vi "NewFile.vi"(8 "error in (no error)":errorcluster, 9 "data flow":T13, 10 "data event in":T17, 11 "config":T22) -> (0 "error out":errorcluster, 2 "data event out":T17, 3 "data event":T1, 4 "registry":T9, 5 "save waveforms":bool)   [LabVIEW 2017, in "McsaDataEventCreator.lvlib"]
uses:
  <vilib>/addons/InsightCM/Devices/Shared/Mcsa/McsaDataEventCreator/McsaDataEventCreator.lvlib
  <vilib>/addons/InsightCM/Devices/Shared/Mcsa/McsaDataEventCreator/controls/config.ctl
  <vilib>/addons/InsightCM/Devices/Shared/Mcsa/McsaDataEventCreator/controls/DataEventConfig.ctl
  <vilib>/addons/InsightCM/Devices/Shared/Mcsa/McsaDataEventCreator/controls/AcqParams.ctl
  <vilib>/addons/InsightCM/Devices/Shared/Common/DataAccumulator/controls/AccumulationSettings.ctl
  <vilib>/addons/InsightCM/Devices/Shared/Common/DataAccumulator/controls/accumulationType.ctl
  <vilib>/addons/InsightCM/Devices/Shared/Common/DVRBuffer/controls/BufferLocation.ctl
  <vilib>/addons/PointValueMap/controls/PointMap.ctl
  <vilib>/addons/InsightCM/Devices/Shared/Common/DataFlow/controls/Data.ctl
  <vilib>/addons/InsightCM/Utilities/DataAccessors/controls/wfmSGL_DVR.ctl
  <vilib>/addons/InsightCM/Devices/Shared/Common/DataFlow/controls/Type.ctl
  <vilib>/addons/InsightCM/Devices/Shared/Mcsa/McsaDataEventCreator/controls/DataGroupRegistry.ctl
  <vilib>/addons/InsightCM/Devices/Shared/Mcsa/McsaDataEventCreator/controls/Registry_DataSet.ctl
  <vilib>/addons/InsightCM/Devices/Shared/Mcsa/McsaDataEventCreator/controls/DataSetType.ctl
  <vilib>/addons/InsightCM/Devices/Shared/Common/DataEventCreator/controls/Registry_Trend.ctl
  <vilib>/addons/InsightCM/Devices/Shared/Common/DataEvent/controls/Event.ctl
  <vilib>/addons/InsightCM/MessageBus/Base/controls/DataEvent.ctl
  <vilib>/addons/InsightCM/MessageBus/Base/controls/KeyValuePair.ctl
  <vilib>/addons/InsightCM/Devices/Shared/Common/DataEvent/controls/DataSet.ctl
  <vilib>/addons/InsightCM/MessageBus/Base/controls/DataSetMetadata.ctl
  <vilib>/addons/InsightCM/MessageBus/Base/controls/TrendPoint.ctl
  <vilib>/addons/InsightCM/MessageBus/Base/controls/TrendAlarmUpdate.ctl
  <vilib>/addons/InsightCM/MessageBus/Base/controls/TrendAlarmTransition.ctl
  <vilib>/addons/InsightCM/Devices/Shared/Common/DataEvent/DataEvent.lvlib
  <vilib>/addons/InsightCM/SRP/SRP.lvlib
  <vilib>/addons/InsightCM/Devices/Shared/Common/DataEventCreator/DataEventCreator.lvlib
  <vilib>/addons/PointValueMap/PointValueMap.lvlib
  <vilib>/addons/InsightCM/Devices/Shared/Common/DataAccumulator/DataAccumulator.lvlib
  <vilib>/addons/InsightCM/Devices/Shared/Common/DVRBuffer/DVRBuffer.lvlib
  <vilib>/addons/InsightCM/Devices/Shared/Common/DataFlow/DataFlow.lvlib
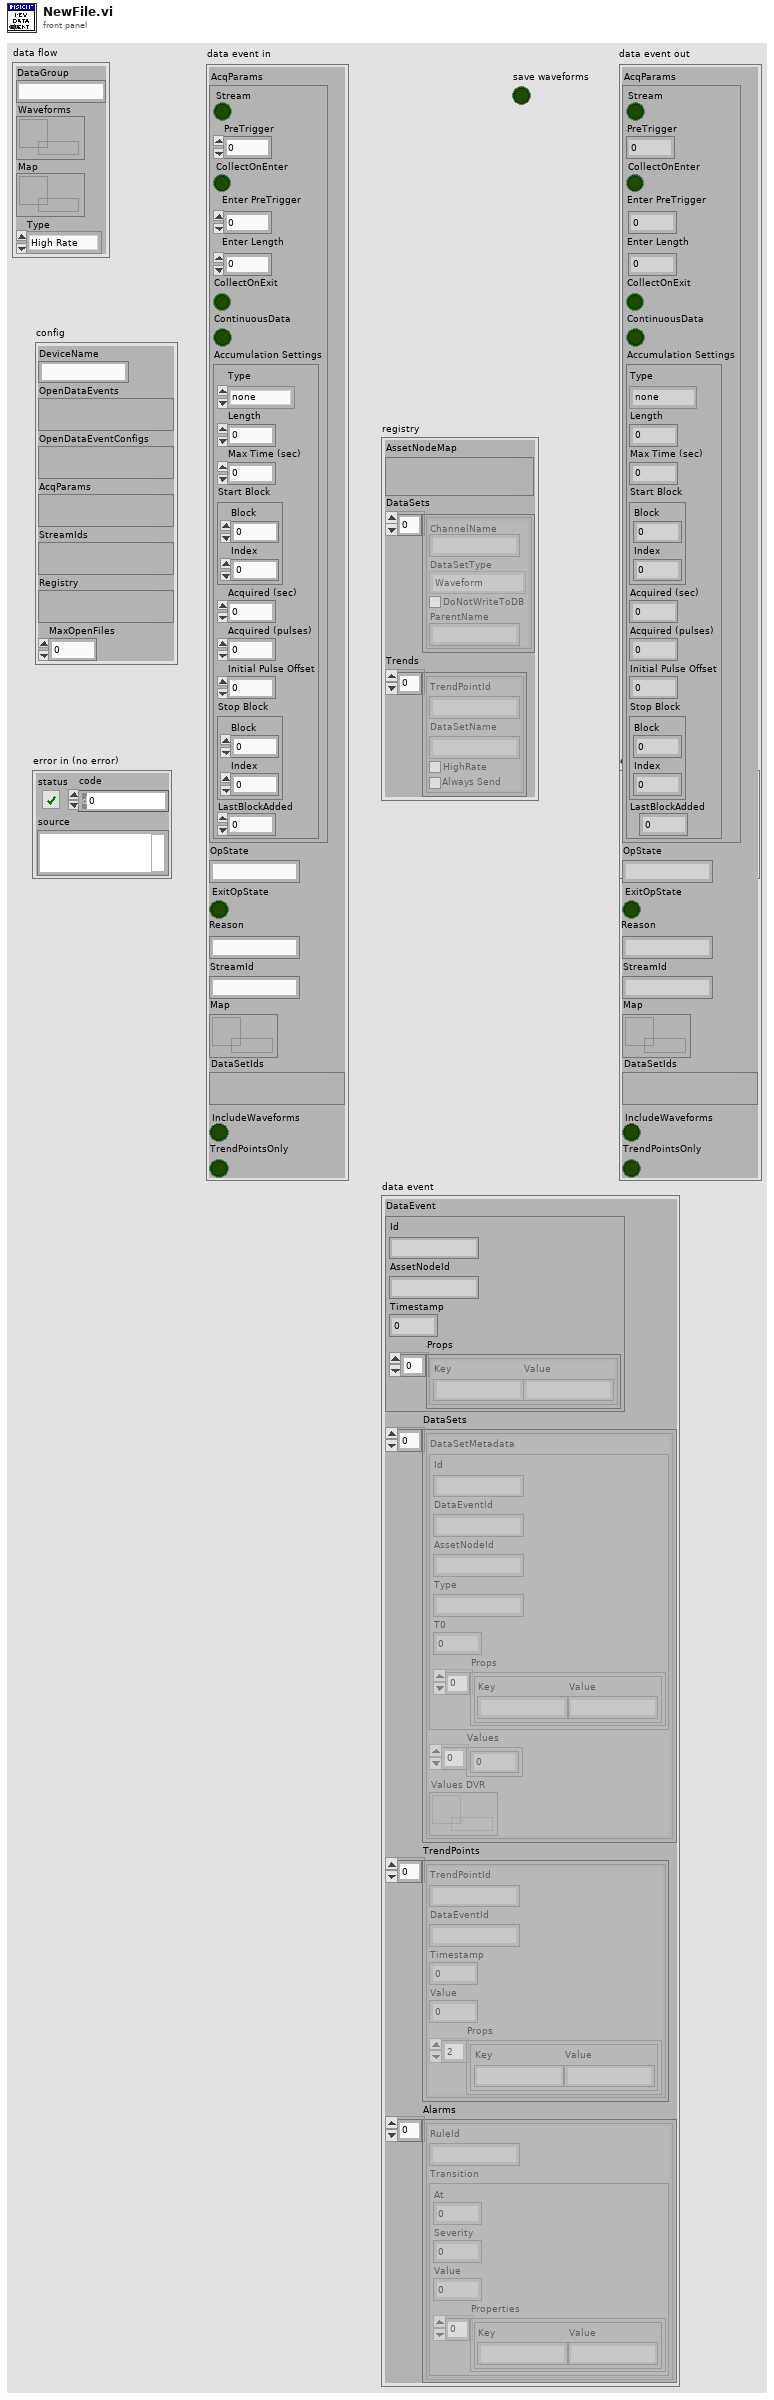
[diagram p1: front panel]
types:
  T1 = typedef "DataEvent.lvlib/Event.ctl" = cluster{"DataEvent":T2, "DataSets":T4[], "TrendPoints":T6[], "Alarms":T7[]}
  T2 = typedef "DataEvent.ctl" = cluster{"Id":string, "AssetNodeId":string, "Timestamp":i64, "Props":T3[]}
  T3 = typedef "KeyValuePair.ctl" = cluster{"Key":string, "Value":string}
  T4 = typedef "DataEvent.lvlib/DataSet.ctl" = cluster{"DataSetMetadata":T5, "Values":sgl[], "Values DVR":refnum<data-value>}
  T5 = typedef "DataSetMetadata.ctl" = cluster{"Id":string, "DataEventId":string, "AssetNodeId":string, "Type":string, "T0":i64, "Props":T3[]}
  T6 = typedef "TrendPoint.ctl" = cluster{"TrendPointId":string, "DataEventId":string, "Timestamp":i64, "Value":dbl, "Props":T3[]}
  T7 = typedef "TrendAlarmUpdate.ctl" = cluster{"RuleId":string, "Transition":T8}
  T8 = typedef "TrendAlarmTransition.ctl" = cluster{"At":i64, "Severity":i32, "Value":dbl, "Properties":T3[]}
  T9 = typedef "McsaDataEventCreator.lvlib/DataGroupRegistry.ctl" = cluster{"AssetNodeMap":variant, "DataSets":T10[], "Trends":T12[]}
  T10 = typedef "McsaDataEventCreator.lvlib/Registry_DataSet.ctl" = cluster{"ChannelName":string, "DataSetType":T11, "DoNotWriteToDB":bool, "ParentName":string}
  T11 = typedef "McsaDataEventCreator.lvlib/DataSetType.ctl" = enum16{"Waveform", "MCSAFFT", "TorqueWFM"}
  T12 = typedef "DataEventCreator.lvlib/Registry_Trend.ctl" = cluster{"TrendPointId":string, "DataSetName":string, "HighRate":bool, "Always Send":bool}
  T13 = typedef "DataFlow.lvlib/Data.ctl" = cluster{"DataGroup":string, "Waveforms":T14, "Map":T15, "Type":T16}
  T14 = typedef "wfmSGL_DVR.ctl" = refnum<data-value>
  T15 = typedef "PointValueMap.lvlib/PointMap.ctl" = refnum<data-value>
  T16 = typedef "DataFlow.lvlib/Type.ctl" = enum16{"High Rate", "Low Rate", "Burst Mode"}
  T17 = typedef "McsaDataEventCreator.lvlib/DataEventConfig.ctl" = cluster{"AcqParams":T18, "OpState":string, "ExitOpState":bool, "Reason":string, "StreamId":string, "Map":T15, "DataSetIds":variant, "IncludeWaveforms":bool, "TrendPointsOnly":bool}
  T18 = typedef "McsaDataEventCreator.lvlib/AcqParams.ctl" = cluster{"Stream":bool, "PreTrigger":i32, "CollectOnEnter":bool, "Enter PreTrigger":i32, "Enter Length":dbl, "CollectOnExit":bool, "ContinuousData":bool, "Accumulation Settings":T19}
  T19 = typedef "DataAccumulator.lvlib/AccumulationSettings.ctl" = cluster{"Type":T20, "Length":dbl, "Max Time (sec)":dbl, "Start Block":T21, "Acquired (sec)":dbl, "Acquired (pulses)":i32, "Initial Pulse Offset":dbl, "Stop Block":T21, "LastBlockAdded":u32}
  T20 = typedef "DataAccumulator.lvlib/accumulationType.ctl" = enum16{"none", "seconds", "revolutions"}
  T21 = typedef "DVRBuffer.lvlib/BufferLocation.ctl" = cluster{"Block":u32, "Index":i32}
  T22 = typedef "McsaDataEventCreator.lvlib/config.ctl" = cluster{"DeviceName":string, "OpenDataEvents":variant, "OpenDataEventConfigs":variant, "AcqParams":variant, "StreamIds":variant, "Registry":variant, "MaxOpenFiles":i32}
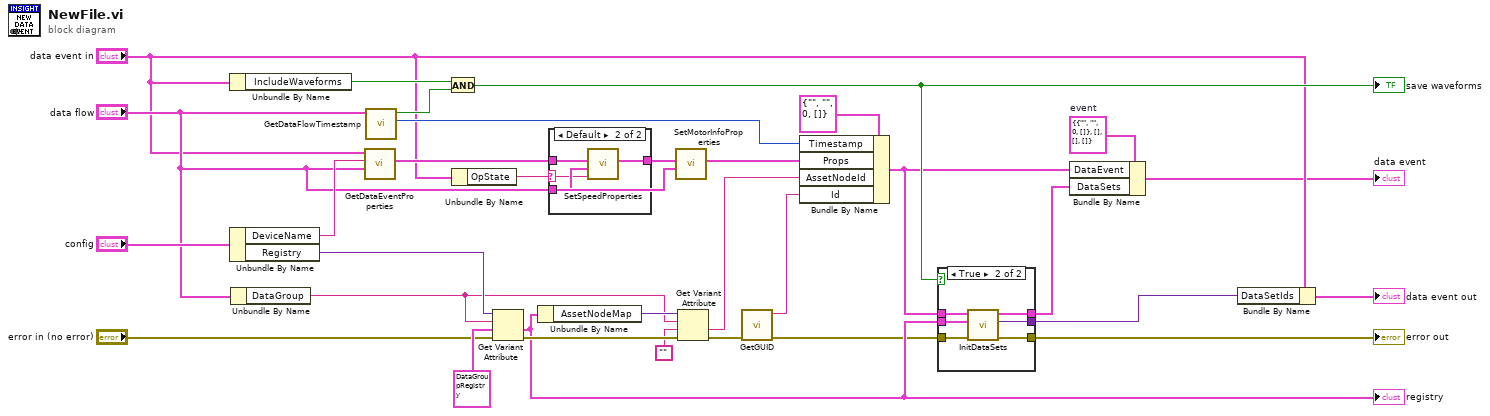
[diagram p0: block diagram]
diagram:
  w29 = T1 {"DataEvent"={"Id"="", "AssetNodeId"="", "Timestamp"=0, "Props"=[]}, "DataSets"=[], "TrendPoints"=[], "Alarms"=[]}  # event
  n1 = Unbundle By Name("data event in") -> ("IncludeWaveforms"=w18:bool)
  n2 = Unbundle By Name("config") -> ("DeviceName"=w17:string, "Registry"=w32:variant)
  n3 = Unbundle By Name("data flow") -> ("DataGroup"=w16:string)
  n4 = call <vilib>:"GetDataEventProperties.vi"("data"="data flow", "device name"=w17, "data event"="data event in") -> ("data event properties"=w8:T3[])  [unwired: 8 in]
  n5 = call <vilib>:"GetDataFlowTimestamp.vi"("data"="data flow") -> ("unix timestamp"=w15:i64, "has waveforms"=w19:bool)  [unwired: 9 in]
  n6 = And(x=w18, y=w19) -> (x .and. y?=w14:bool)
  "save waveforms" <- w14
  n7 = Unbundle By Name("data event in") -> ("OpState"=w4:string)
  n8 = Get Variant Attribute(Variant=w32, name=w16, default value (empty Variant)=T9 {"AssetNodeMap"=variant, "DataSets"=[], "Trends"=[]} ("Data Group Registry"), error in="error in (no error)") -> (value=w13:T9, error out=w25:errorcluster)  [unwired: 2 out]
  "registry" <- w13
  n9 = Unbundle By Name(w13) -> ("AssetNodeMap"=w26:variant)
  n10 = case shown="Default" w4 {
    selector: w4 -> [_ w34]
    tunnel: w8 -> [w33 w37]
    tunnel: [w33 w36] -> w7
    tunnel: "data flow" -> [_ w35]
    frame "Startup" {
    }
    frame Default {
      n11 = call <vilib>:"SetSpeedProperties.vi"("OpState"=w34, "data"=w35, "data event properties in"=w37) -> ("data event properties out"=w36:T3[])  [unwired: 8 in]
    }
  }
  n12 = call <vilib>:"SetMotorInfoProperties.vi"("data"="data flow", "data event properties in"=w7) -> ("data event properties out"=w6:T3[])  [unwired: 9 in]
  n13 = Get Variant Attribute(Variant=w26, name=w16, default value (empty Variant)="", error in=w25) -> (value=w23:string, error out=w20:errorcluster)  [unwired: 2 out]
  n14 = call <vilib>:"GetGUID.vi"("error in (no error)"=w20) -> ("error out"=w12:errorcluster, "GUID"=w22:string)  [unwired: 9 in]
  n15 = Bundle By Name(cluster=T2 {"Id"="", "AssetNodeId"="", "Timestamp"=0, "Props"=[]} ("DataEvent"), "Timestamp"=w15, "Props"=w6, "AssetNodeId"=w23, "Id"=w22) -> (w9:T2)
  n16 = case shown="True" w14 {
    tunnel: w13 -> [_ w40]
    tunnel: w12 -> [w38 w44]
    tunnel: [_ w43] -> w11
    tunnel: [w38 w42] -> w2
    tunnel: [_ w41] -> w10
    tunnel: w9 -> [_ w39]
    frame False {
    }
    frame True {
      n17 = call <vilib>:"InitDataSets.vi"("error in (no error)"=w44, "registry"=w40, "dataevent"=w39) -> ("error out"=w42:errorcluster, "datasetIds"=w43:variant, "datasets"=w41:T4[])  [unwired: 6 in]
    }
  }
  "error out" <- w2
  n18 = Bundle By Name(cluster=w29, "DataEvent"=w9, "DataSets"=w10) -> (→"data event":T1)
  n19 = Bundle By Name(cluster="data event in", "DataSetIds"=w11) -> (→"data event out":T17)
